vi "Initialization VI.vi"(8 "error in (no error)":errorcluster, 10 "Custom XML":string, 11 "Device Item Ref in":T1 format="%.0x") -> (0 "error out":errorcluster, 3 "Device Item Ref out":T1 format="%.0x")   [LabVIEW 2025, in "Protection and Counter Addon System Explorer.lvlib"]
uses:
  Protection and Counter Addon System Explorer.lvlib
  <vilib>/NI VeriStand/Custom Device API/Custom Device Item Ref.ctl
  <vilib>/NI VeriStand/Custom Device Tools/Custom Device Utility Library/Search Direction.ctl
  <vilib>/NI VeriStand/Custom Device API/Custom Device Channel.ctl
  <vilib>/NI VeriStand/Custom Device API/Custom Device Channel Type.ctl
  Addon Shared/SubVIs/GUID Lookup.vi
  <vilib>/NI VeriStand/Custom Device Tools/Custom Device Utility Library/NI VeriStand - Search for Item by GUID.vi
  <vilib>/NI VeriStand/Custom Device API/Custom Device API.lvlib
  Addon Shared/Protection and Counter Addon Shared.lvlib
  <vilib>/NI/NI VeriStand Custom Device Import and Export Tool/ImportExport.lvlib
  <vilib>/NI VeriStand/Custom Device Tools/Custom Device Utility Library/Custom Device Utility Library.lvlib
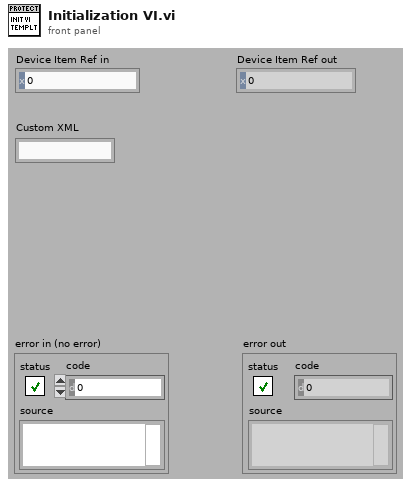
[diagram p1: front panel]
types:
  T1 = typedef "Custom Device API.lvlib/Custom Device Item Ref.ctl" = u64
  T2 = typedef "Custom Device Utility Library.lvlib/Search Direction.ctl" = enum16{"Down", "Up"}
  T3 = typedef "Custom Device API.lvlib/Custom Device Channel.ctl" = cluster{"Type":T4, "Units":string, "Default Value":dbl, "Faultable":bool, "Scalable":bool}
  T4 = typedef "Custom Device API.lvlib/Custom Device Channel Type.ctl" = enum16{"Input", "Output"}
  T5 = typedef "Protection and Counter Addon Shared.lvlib/XNET Settings.ctl" = cluster{"Database":refnum<k21>, "Cluster":refnum<k21>, "Port":string, "Baud rate [Bd]":u64, "Termination":u32, "CAN I/O Mode":u32, "FD Baud rate [Bd]":u64, "Priority":i32, "Use Legacy":bool, "FD ISO Mode":u32, "Default Max Counter Value":dbl, "Default Protect Type":T6, "Include All Channels":bool}
  T6 = typedef "Protection and Counter Support Shared.lvlib/Protection Type.ctl" = enum16{"Arb ID + Bytes Checksum with Inversion", "Arb ID + Bytes CRC with Inversion", "Reversed Raw Signal Checksum with Inversion", "Concatenated Two's Compliment"}
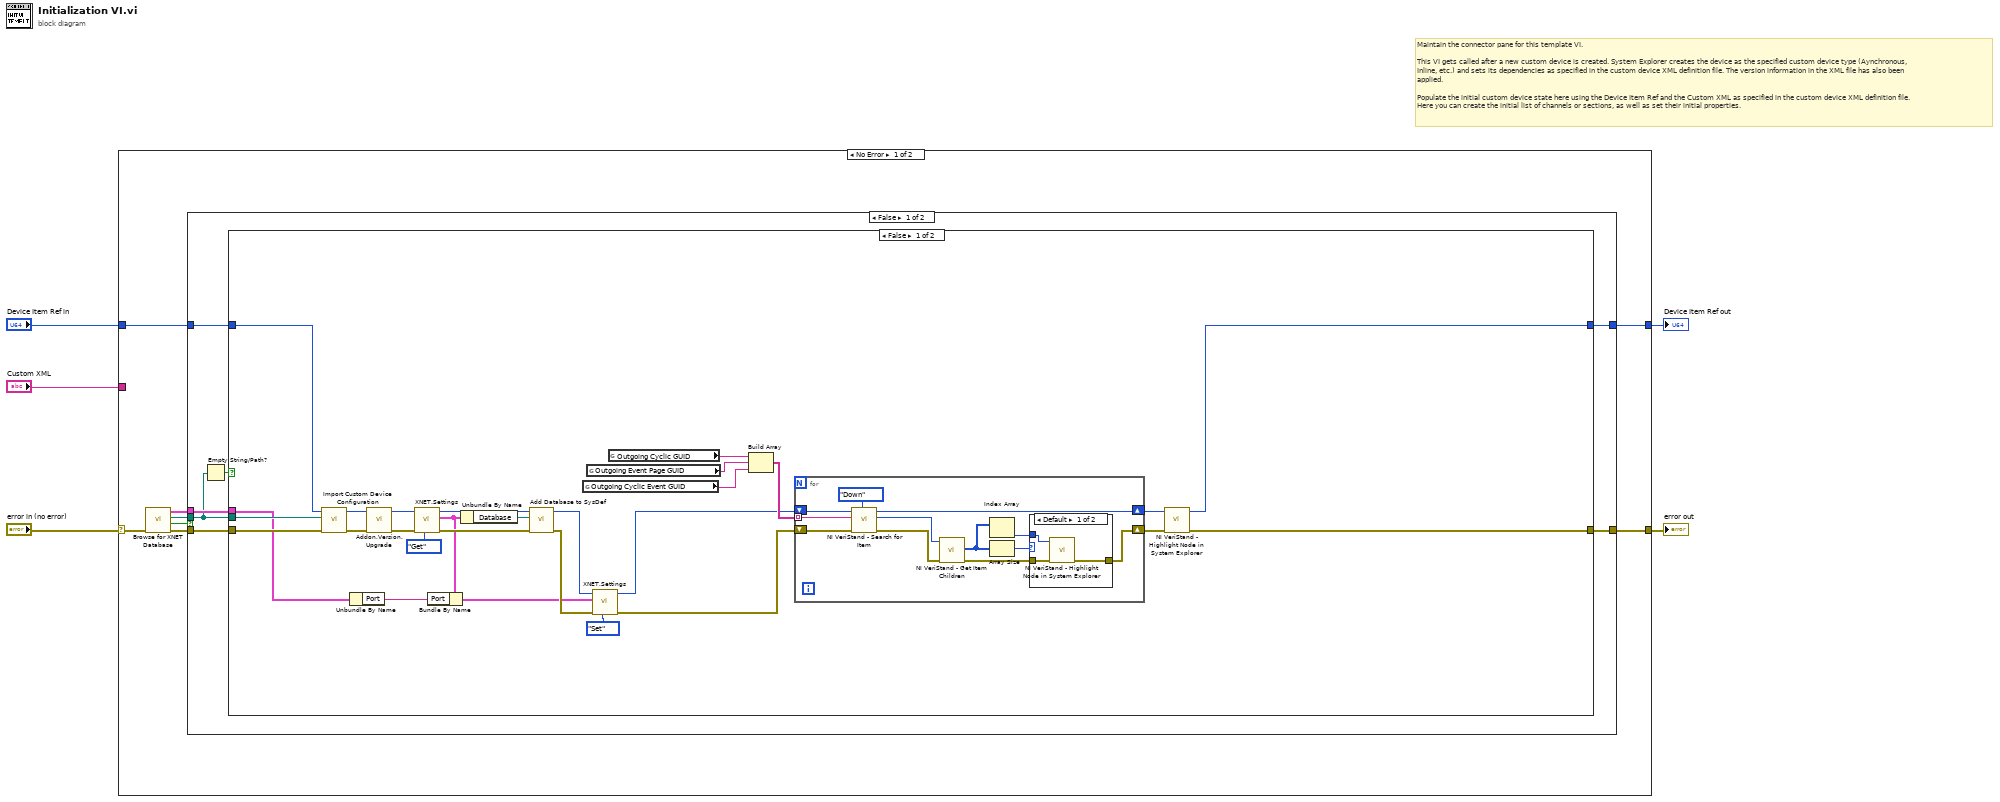
[diagram p0: block diagram]
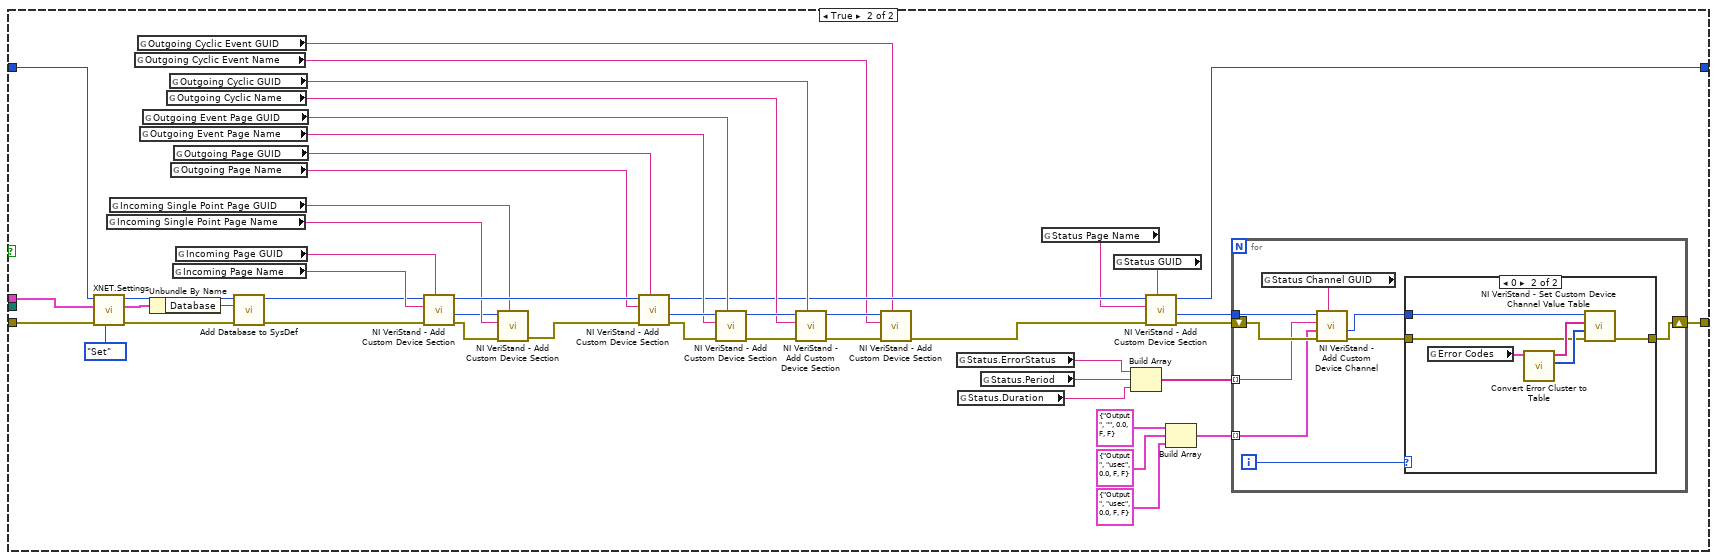
[diagram p3: hidden frame]
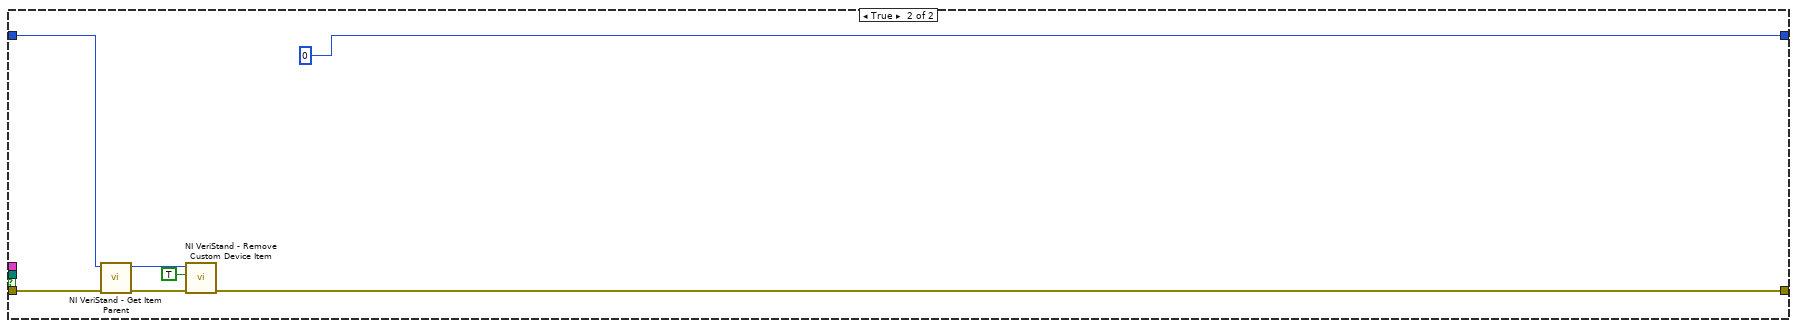
[diagram p5: hidden frame]
diagram:
  # "Maintain the connector pane for this template VI.\n\nThis VI gets called after a new custom device is created. System Explorer creates the device as the specified custom device type (Aynchronous, Inline, etc.) and sets its dependencies as specified in the custom device XML definition file. The version information in the XML file has also been applied.\n\nPopulate the initial custom device state here using the Device Item Ref and the Custom XML as specified in the custom device XML definition file. Here you can create the initial list of channels or sections, as well as set their initial properties."
  n1 = case shown="No Error" "error in (no error)" {
    selector: "error in (no error)" -> [w11 w137]
    tunnel: [w13 w137] -> w5
    tunnel: [w12 w136] -> w3
    tunnel: "Device Item Ref in" -> [w9 w136]
    tunnel: "Custom XML" -> [_ _]
    frame No Error {
      n2 = call "Browse for XNET Database.vi"("error in (no error)"=w11) -> ("error out"=w10:errorcluster, "Cancel Out"=w7:bool, "Import Path out"=w6:path, "XNET Settings"=w8:T5)  [unwired: 7 in]
      n3 = case shown="False" w7 {
        tunnel: [w16 w130] -> w13
        tunnel: [w17 T1 0 ("Parent Ref out")] -> w12
        tunnel: w10 -> [w20 w133]
        tunnel: w9 -> [w19 w135]
        tunnel: w8 -> [w18 _]
        tunnel: w6 -> [w14 _]
        frame False {
          n4 = Empty String/Path?(string/path=w14) -> (empty?=w15:bool)
          n5 = case shown="False" w15 {
            tunnel: w20 -> [w29 w105]
            tunnel: w19 -> [w48 w103]
            tunnel: w18 -> [w22 w101]
            tunnel: [w38 w83] -> w17
            tunnel: [w37 w82] -> w16
            tunnel: w14 -> [w47 _]
            frame False {
              n6 = call <vilib>:"Import Custom Device Configuration.vi"("error in (no error)"=w29, "Path"=w47, "NodeID"=w48) -> ("error out"=w46:errorcluster, "NodeID out"=w45:u64)  [unwired: 6 in, 1 out]
              n7 = Unbundle By Name(w22) -> ("Port"=w21:string)
              n8 = call "Addon.Version.Upgrade.vi"("error in (no error)"=w46, "Device Item Ref in in"=w45) -> ("error out"=w43:errorcluster, "Device Item Ref out"=w41:T1)  [unwired: 8 in]
              n9 = call "XNET.Settings.vi"("Action"=enum8{"Get", "Set"}."Get", "error in (no error)"=w43, "Parent Ref in"=w41) -> ("error out"=w42:errorcluster, "XNET Settings"=w27:T5, "Item Ref out"=w40:T1)  [unwired: 6 in]
              n10 = Bundle By Name(cluster=w27, "Port"=w21) -> (w26:T5)
              n11 = Unbundle By Name(w27) -> ("Database"=w39:refnum<k21>)
              n12 = call "Add Database to SysDef.vi"("error in"=w42, "DB Alias"=w39, "Item Ref in"=w40) -> ("error out"=w28:errorcluster, "Item Ref out"=w24:T1)  [unwired: 7 in]
              n13 = global read "GUID Lookup.vi" "Outgoing Cyclic Event GUID"() -> (w34:string)
              n14 = global read "GUID Lookup.vi" "Outgoing Event Page GUID"() -> (w35:string)
              n15 = call "XNET.Settings.vi"("Action"=enum8{"Get", "Set"}."Set", "error in (no error)"=w28, "XNET Settings"=w26, "Parent Ref in"=w24) -> ("error out"=w25:errorcluster, "Item Ref out"=w23:T1)  [unwired: 5 in, 1 out]
              n16 = global read "GUID Lookup.vi" "Outgoing Cyclic GUID"() -> (w36:string)
              n17 = Build Array(w36, w35, w34) -> (w33:string[])
              n18 = for {
                tunnel: w33 -> [w58] mode=indexing
                shift-right: [w49] -> w32
                shift-left: w25 -> [w57]
                shift-right: [w56] -> w31
                shift-left: w23 -> [w59]
                n19 = call-poly <vilib>:"NI VeriStand - Search for Item.vi"("Direction (Down)"=Search_Direction."Down", "error in"=w57, "Item GUID"=w58, "Section Ref in"=w59) -> ("error out"=w54:errorcluster, "Item Ref"=w55:T1, "Section Ref out"=w56:T1)  [unwired: 4 in, 1 out]
                n20 = call <vilib>:"NI VeriStand - Get Item Children.vi"("error in (no error)"=w54, "Item Ref in"=w55) -> ("error out"=w50:errorcluster, "Child Refs"=w52:T1[])  [unwired: 6 in, 2 out]
                n21 = Index Array(array=w52) -> (element=w51:T1)  [unwired: 1 in]
                n22 = Array Size(array=w52) -> (size(s)=w53:i32)
                n23 = case shown="Default" w53 {
                  tunnel: w51 -> [w63 _]
                  tunnel: w50 -> [w62 w64]
                  tunnel: [w61 w64] -> w49
                  frame Default {
                    n24 = call <vilib>:"NI VeriStand - Highlight Node in System Explorer.vi"("error in (no error)"=w62, "Item Ref in"=w63) -> ("error out"=w61:errorcluster)  [unwired: 8 in, 1 out]
                  }
                  frame -1, 0 {
                  }
                }
              }
              n25 = call <vilib>:"NI VeriStand - Highlight Node in System Explorer.vi"("error in (no error)"=w32, "Item Ref in"=w31) -> ("error out"=w37:errorcluster, "Node Ptr dup"=w38:T1)  [unwired: 8 in]
            }
            frame True {
              n26 = call "XNET.Settings.vi"("Action"=enum8{"Get", "Set"}."Set", "error in (no error)"=w105, "XNET Settings"=w101, "Parent Ref in"=w103) -> ("error out"=w104:errorcluster, "XNET Settings"=w100:T5, "Item Ref out"=w102:T1)  [unwired: 5 in]
              n27 = global read "GUID Lookup.vi" "Incoming Single Point Page Name"() -> (w87:string)
              n28 = global read "GUID Lookup.vi" "Incoming Single Point Page GUID"() -> (w88:string)
              n29 = global read "GUID Lookup.vi" "Outgoing Cyclic Event Name"() -> (w71:string)
              n30 = global read "GUID Lookup.vi" "Outgoing Cyclic Event GUID"() -> (w72:string)
              n31 = global read "GUID Lookup.vi" "Outgoing Event Page Name"() -> (w92:string)
              n32 = global read "GUID Lookup.vi" "Outgoing Event Page GUID"() -> (w93:string)
              n33 = Unbundle By Name(w100) -> ("Database"=w99:refnum<k21>)
              n34 = global read "GUID Lookup.vi" "Outgoing Cyclic Name"() -> (w90:string)
              n35 = global read "GUID Lookup.vi" "Outgoing Cyclic GUID"() -> (w91:string)
              n36 = global read "GUID Lookup.vi" "Outgoing Page Name"() -> (w109:string)
              n37 = global read "GUID Lookup.vi" "Incoming Page Name"() -> (w108:string)
              n38 = global read "GUID Lookup.vi" "Outgoing Page GUID"() -> (w110:string)
              n39 = global read "GUID Lookup.vi" "Incoming Page GUID"() -> (w112:string)
              n40 = call "Add Database to SysDef.vi"("error in"=w104, "DB Alias"=w99, "Item Ref in"=w102) -> ("error out"=w107:errorcluster, "Item Ref out"=w106:T1)  [unwired: 7 in]
              n41 = call <vilib>:"NI VeriStand - Add Custom Device Section.vi"("GUID (Default Section)"=w112, "error in (no error)"=w107, "Section Name"=w108, "Parent Ref in"=w106) -> ("error out"=w65:errorcluster, "Section Ptr"=w66:T1, "Parent Ref out"=w111:T1)  [unwired: 4 in, 1 out]
              n42 = call <vilib>:"NI VeriStand - Add Custom Device Section.vi"("GUID (Default Section)"=w88, "error in (no error)"=w65, "Section Name"=w87, "Parent Ref in"=w66) -> ("error out"=w89:errorcluster)  [unwired: 4 in, 3 out]
              n43 = call <vilib>:"NI VeriStand - Add Custom Device Section.vi"("GUID (Default Section)"=w110, "error in (no error)"=w89, "Section Name"=w109, "Parent Ref in"=w111) -> ("error out"=w95:errorcluster, "Section Ptr"=w97:T1, "Parent Ref out"=w84:T1)  [unwired: 4 in, 1 out]
              n44 = call <vilib>:"NI VeriStand - Add Custom Device Section.vi"("GUID (Default Section)"=w93, "error in (no error)"=w95, "Section Name"=w92, "Parent Ref in"=w97) -> ("error out"=w96:errorcluster, "Parent Ref out"=w94:T1)  [unwired: 4 in, 2 out]
              n45 = call <vilib>:"NI VeriStand - Add Custom Device Section.vi"("GUID (Default Section)"=w91, "error in (no error)"=w96, "Section Name"=w90, "Parent Ref in"=w94) -> ("error out"=w74:errorcluster, "Parent Ref out"=w75:T1)  [unwired: 4 in, 2 out]
              n46 = call <vilib>:"NI VeriStand - Add Custom Device Section.vi"("GUID (Default Section)"=w72, "error in (no error)"=w74, "Section Name"=w71, "Parent Ref in"=w75) -> ("error out"=w73:errorcluster)  [unwired: 4 in, 3 out]
              n47 = global read "GUID Lookup.vi" "Status.ErrorStatus"() -> (w81:string)
              n48 = global read "GUID Lookup.vi" "Status.Duration"() -> (w79:string)
              n49 = global read "GUID Lookup.vi" "Status.Period"() -> (w80:string)
              n50 = global read "GUID Lookup.vi" "Status Page Name"() -> (w76:string)
              n51 = global read "GUID Lookup.vi" "Status GUID"() -> (w77:string)
              n52 = Build Array(w81, w80, w79) -> (w78:string[])
              n53 = call <vilib>:"NI VeriStand - Add Custom Device Section.vi"("GUID (Default Section)"=w77, "error in (no error)"=w73, "Section Name"=w76, "Parent Ref in"=w84) -> ("error out"=w85:errorcluster, "Section Ptr"=w86:T1, "Parent Ref out"=w83:T1)  [unwired: 4 in, 1 out]
              n54 = Build Array(T3 {"Type"=enum."Output", "Units"="", "Default Value"=0.0, "Faultable"=FALSE, "Scalable"=FALSE} ("Channel"), T3 {"Type"=enum."Output", "Units"="usec", "Default Value"=0.0, "Faultable"=FALSE, "Scalable"=FALSE} ("Channel"), T3 {"Type"=enum."Output", "Units"="usec", "Default Value"=0.0, "Faultable"=FALSE, "Scalable"=FALSE} ("Channel")) -> (w67:T3[])
              n55 = for {
                tunnel: w86 -> [w121]
                shift-right: [w114] -> w82
                shift-left: w85 -> [w120]
                tunnel: w78 -> [w118] mode=indexing
                tunnel: w67 -> [w117] mode=indexing
                i -> [w116]
                n56 = global read "GUID Lookup.vi" "Status Channel GUID"() -> (w119:string)
                n57 = call <vilib>:"NI VeriStand - Add Custom Device Channel.vi"("GUID (Default Channel)"=w119, "error in (no error)"=w120, "Channel"=w117, "Channel Name"=w118, "Parent Ref in"=w121) -> ("error out"=w115:errorcluster, "Channel Ref"=w113:T1)  [unwired: 3 in, 2 out]
                n58 = case shown="0" w116 {
                  tunnel: w113 -> [_ w127]
                  tunnel: w115 -> [w122 w124]
                  tunnel: [w122 w123] -> w114
                  frame Default {
                  }
                  frame 0 {
                    n59 = global read "GUID Lookup.vi" "Error Codes"() -> (w128:cluster{"number":i32, "trimmed string":string}[])
                    n60 = call "Convert Error Cluster to Table.vi"("Error Codes"=w128) -> ("Code"=w125:i32[], "String"=w126:string[])  [unwired: 9 in]
                    n61 = call <vilib>:"NI VeriStand - Set Custom Device Channel Value Table.vi"("error in (no error)"=w124, "Values"=w125, "Names"=w126, "Channel Ref in"=w127) -> ("error out"=w123:errorcluster)  [unwired: 6 in, 1 out]
                  }
                }
              }
            }
          }
        }
        frame True {
          n62 = call <vilib>:"NI VeriStand - Get Item Parent.vi"("error in (no error)"=w133, "Item Ref in"=w135) -> ("error out"=w134:errorcluster, "Item Ref out"=w132:T1)  [unwired: 6 in, 2 out]
          n63 = call <vilib>:"NI VeriStand - Remove Custom Device Item.vi"("error in (no error)"=w134, "Force Delete (F)"=TRUE, "Item Ref in"=w132) -> ("error out"=w130:errorcluster)  [unwired: 7 in, 1 out]
        }
      }
    }
    frame Error {
    }
  }
  "error out" <- w5
  "Device Item Ref out" <- w3
